vi "carwash_test2_mod.vi"() -> ()   [LabVIEW 2017]
panel:
  out "Enum":enum16{""}(ring)
  out "number":u32
  out "x+y":i32
  out "x*y":i32
  out "output cluster":cluster{bool, bool}
  in  "Economy Wash":bool
  in  "Deluxe Wash":bool
  in  "?":bool
  in  "Wash Select":enum16{"Initialize", "Deluxe", "Economy"}(ring)
  out "Vehicle Out of Position":bool=TRUE
  out "Air Dry":bool
  out "Clear Water Rinse":bool
  out "Main High Press. Wash":bool
  out "Soap Application":bool
  out "Under body Wash":bool
  in  "?":bool
  in  "0":bool
  in  "stop":bool
  # "Car Wash Indicators"
  # "Underbody wash\nposition \nSwitch"
  # "Main Wash \nPosition \nSwitch"
  # "Air Dry\nPosition\nSwitch"
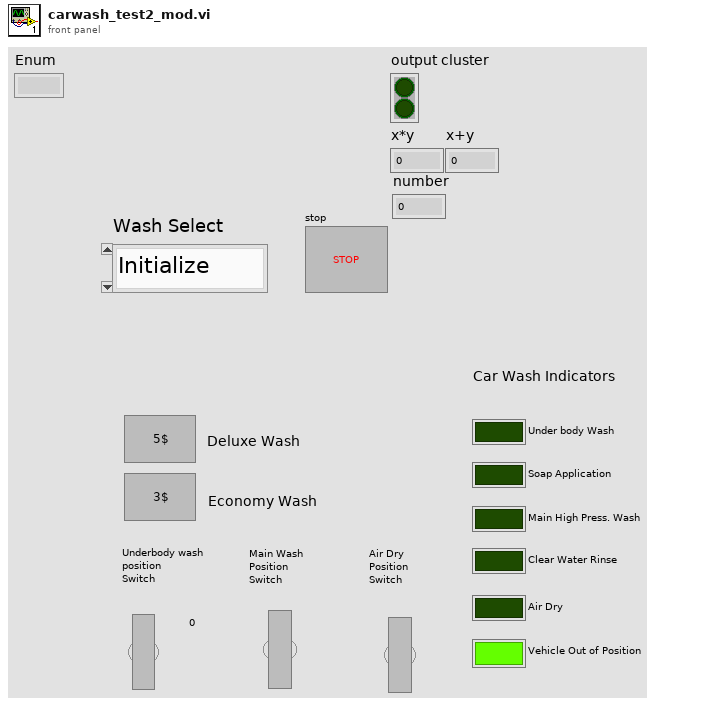
[diagram p1: front panel]
types:
  T1 = enum8{"Enabled", "Disabled", "Disabled and Grayed Out"}
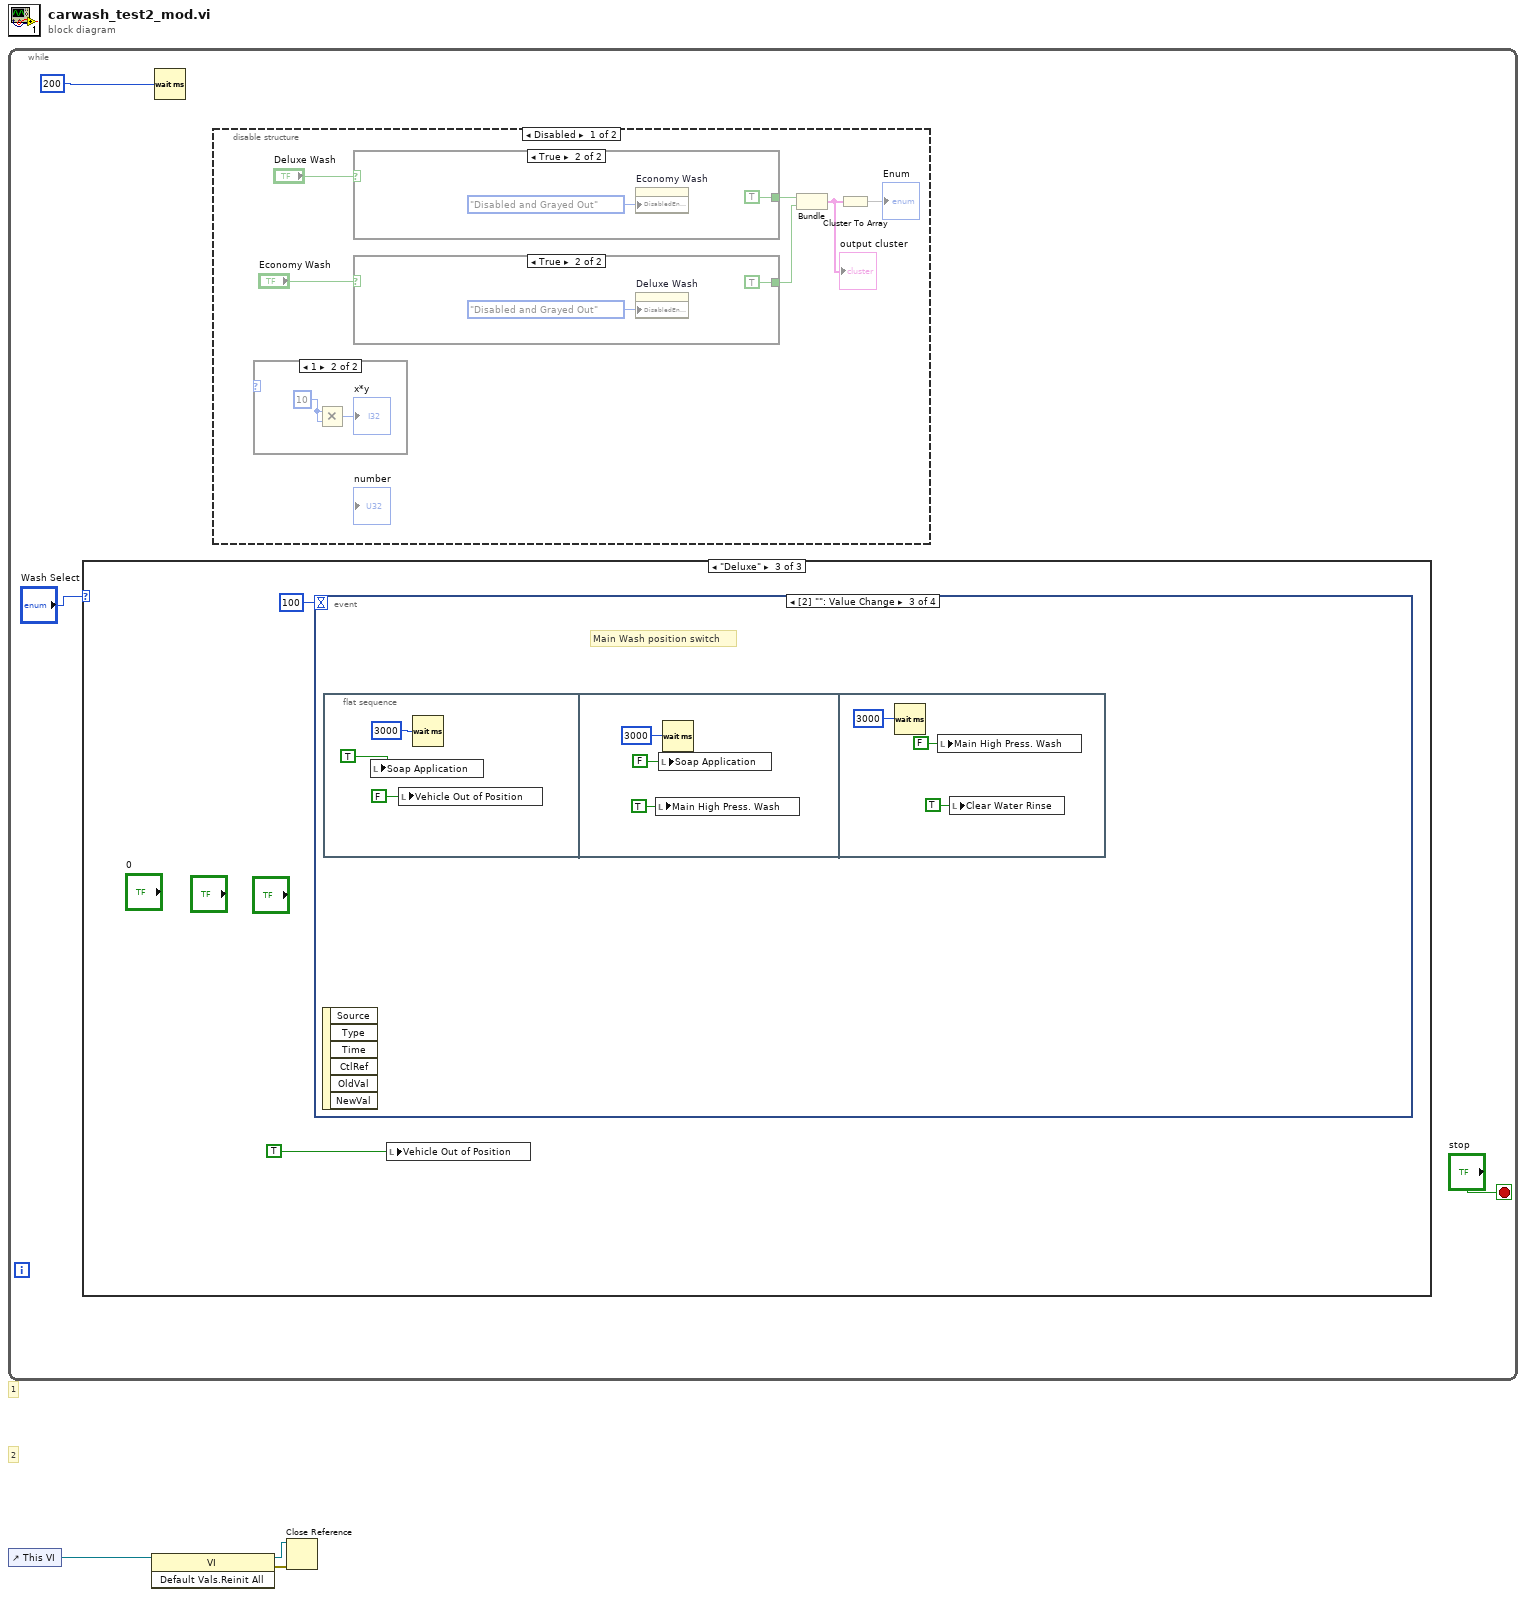
[diagram p0: block diagram]
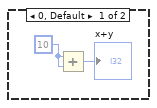
[diagram p2: hidden frame]
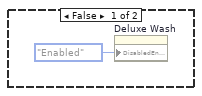
[diagram p3: hidden frame]
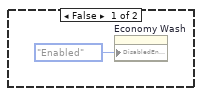
[diagram p4: hidden frame]
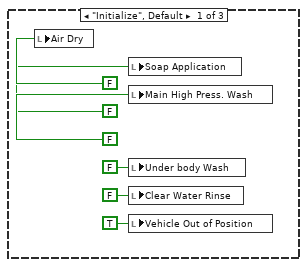
[diagram p6: hidden frame]
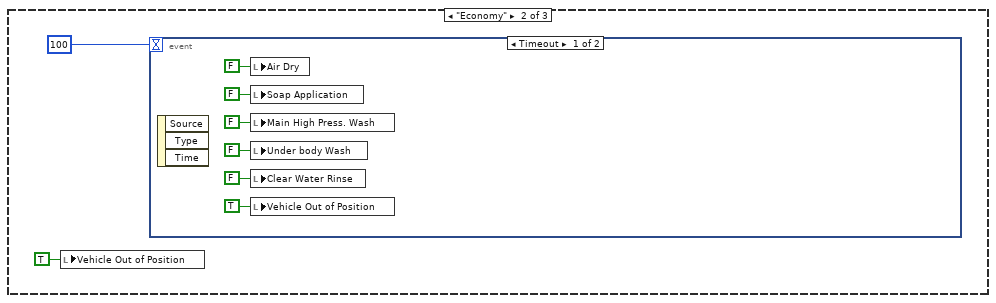
[diagram p7: hidden frame]
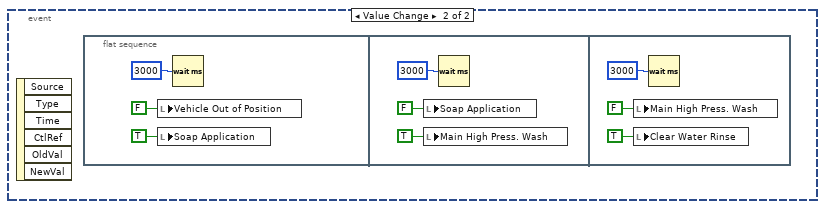
[diagram p8: hidden frame]
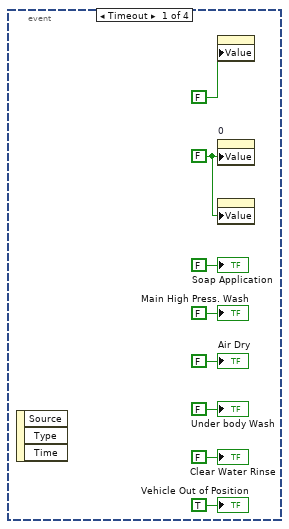
[diagram p9: hidden frame]
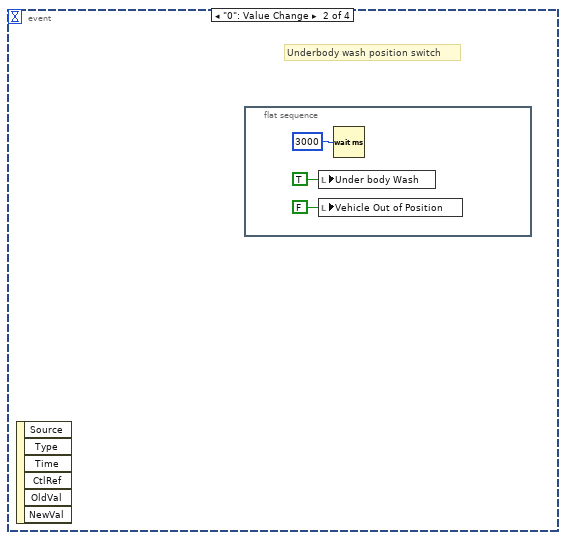
[diagram p10: hidden frame]
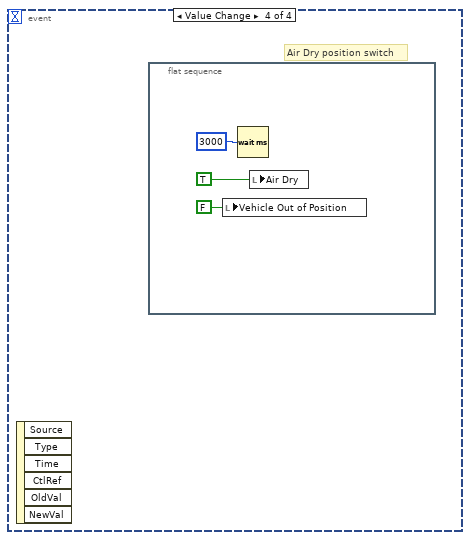
[diagram p11: hidden frame]
diagram:
  # "1"
  # "2"
  n1 = while {
    stop <- "stop" stop-if-true
    n2 = case shown="\"Deluxe\"" "Wash Select" {
      frame "Initialize", Default {
        n3 = local write "Air Dry"(FALSE) -> ()
        n4 = local write "Soap Application"(FALSE) -> ()
        n5 = local write "Main High Press. Wash"(FALSE) -> ()
        n6 = local write "Under body Wash"(FALSE) -> ()
        n7 = local write "Clear Water Rinse"(FALSE) -> ()
        n8 = local write "Vehicle Out of Position"(TRUE) -> ()
      }
      frame "Economy" {
        n9 = local write "Vehicle Out of Position"(TRUE ("Vehicle Out of Position")) -> ()
        n10 = event shown="[0] Timeout" {
          selector: _ -> [_ _]
          dyn-events: _ -> [_ _]
          timeout: 100 -> [_ _]
          event Timeout {
            n11 = event-data() -> ()  [unwired: 1 in, 3 out]
            n12 = local write "Air Dry"(FALSE) -> ()
            n13 = local write "Soap Application"(FALSE) -> ()
            n14 = local write "Main High Press. Wash"(FALSE) -> ()
            n15 = local write "Under body Wash"(FALSE) -> ()
            n16 = local write "Clear Water Rinse"(FALSE) -> ()
            n17 = local write "Vehicle Out of Position"(TRUE ("Vehicle Out of Position")) -> ()
          }
          event Value Change {
            n18 = event-data() -> ()  [unwired: 1 in, 6 out]
            n19 = flat-sequence {
              frame #0 {
                n20 = local write "Vehicle Out of Position"(FALSE ("Vehicle Out of Position")) -> ()
                n21 = local write "Soap Application"(TRUE ("Soap Application")) -> ()
                n22 = Wait (ms)(milliseconds to wait=u32 3000) -> ()  [unwired: 1 out]
              }
              frame #1 {
                n23 = local write "Soap Application"(FALSE ("Soap Application")) -> ()
                n24 = local write "Main High Press. Wash"(TRUE ("Main High Press. Wash")) -> ()
                n25 = Wait (ms)(milliseconds to wait=u32 3000) -> ()  [unwired: 1 out]
              }
              frame #2 {
                n26 = local write "Main High Press. Wash"(FALSE ("Main High Press. Wash")) -> ()
                n27 = local write "Clear Water Rinse"(TRUE ("Clear Water Rinse")) -> ()
                n28 = Wait (ms)(milliseconds to wait=u32 3000) -> ()  [unwired: 1 out]
              }
            }
          }
        }
      }
      frame "Deluxe" {
        n29 = event shown="[2] \"\": Value Change" {
          selector: _ -> [_ _ _ _]
          dyn-events: _ -> [_ _ _ _]
          timeout: 100 -> [_ _ _ _]
          event Timeout {
            w55 = FALSE
            n30 = event-data() -> ()  [unwired: 1 in, 3 out]
            n31 = property class="Bool (strict)"("Value"=FALSE) -> ()  [unwired: 2 in, 2 out]
            n32 = property on="0" class="Bool (strict)"("Value"=w55) -> ()  [unwired: 2 in, 2 out]
            n33 = property class="Bool (strict)"("Value"=w55) -> ()  [unwired: 2 in, 2 out]
            "Air Dry" <- FALSE
            "Vehicle Out of Position" <- TRUE
            "Clear Water Rinse" <- FALSE
            "Under body Wash" <- FALSE
            "Main High Press. Wash" <- FALSE
            "Soap Application" <- FALSE
          }
          event "0": Value Change {
            # "Underbody wash position switch"
            n34 = event-data() -> ()  [unwired: 1 in, 6 out]
            n35 = flat-sequence {
              frame #0 {
                n36 = local write "Under body Wash"(TRUE ("Under body Wash")) -> ()
                n37 = local write "Vehicle Out of Position"(FALSE ("Vehicle Out of Position")) -> ()
                n38 = Wait (ms)(milliseconds to wait=u32 3000) -> ()  [unwired: 1 out]
              }
            }
          }
          event Value Change {
            # "Main Wash position switch"
            n39 = event-data() -> ()  [unwired: 1 in, 6 out]
            n40 = flat-sequence {
              frame #0 {
                n41 = local write "Soap Application"(TRUE ("Air Dry")) -> ()
                n42 = local write "Vehicle Out of Position"(FALSE ("Vehicle Out of Position")) -> ()
                n43 = Wait (ms)(milliseconds to wait=u32 3000) -> ()  [unwired: 1 out]
              }
              frame #1 {
                n44 = local write "Main High Press. Wash"(TRUE ("Main High Press. Wash")) -> ()
                n45 = local write "Soap Application"(FALSE ("Under body Wash")) -> ()
                n46 = Wait (ms)(milliseconds to wait=u32 3000) -> ()  [unwired: 1 out]
              }
              frame #2 {
                n47 = Wait (ms)(milliseconds to wait=u32 3000) -> ()  [unwired: 1 out]
                n48 = local write "Main High Press. Wash"(FALSE ("Main High Press. Wash")) -> ()
                n49 = local write "Clear Water Rinse"(TRUE ("Clear Water Rinse")) -> ()
              }
            }
          }
          event Value Change {
            # "Air Dry position switch"
            n50 = event-data() -> ()  [unwired: 1 in, 6 out]
            n51 = flat-sequence {
              frame #0 {
                n52 = local write "Vehicle Out of Position"(FALSE ("Vehicle Out of Position")) -> ()
                n53 = Wait (ms)(milliseconds to wait=u32 3000) -> ()  [unwired: 1 out]
                n54 = local write "Air Dry"(TRUE ("Boolean 2")) -> ()
              }
            }
          }
        }
        n55 = local write "Vehicle Out of Position"(TRUE ("Vehicle Out of Position")) -> ()
      }
    }
    n56 = Wait (ms)(milliseconds to wait=u32 200) -> ()  [unwired: 1 out]
    n57 = disable-structure shown="Disabled" {
      frame Disabled {
        n58 = case shown="1" {
          selector: _ -> [_ _]
          frame 0, Default {
            w14 = 10
            n59 = Add(x=w14, y=w14) -> (x+y=→"x+y":i32)
          }
          frame 1 {
            w16 = 10
            n60 = Multiply(x=w16, y=w16) -> (x*y=→"x*y":i32)
          }
        }
        n61 = case shown="True" "Deluxe Wash" {
          tunnel: [_ TRUE] -> w10
          frame False {
            n62 = property on="Economy Wash" class="Bool (strict)"("DisabledEnum"=T1."Enabled" ("Disabled")) -> ()  [unwired: 2 in, 2 out]
          }
          frame True {
            n63 = property on="Economy Wash" class="Bool (strict)"("DisabledEnum"=T1."Disabled and Grayed Out" ("Disabled")) -> ()  [unwired: 2 in, 2 out]
          }
        }
        n64 = case shown="True" "Economy Wash" {
          tunnel: [_ TRUE] -> w9
          frame False {
            n65 = property on="Deluxe Wash" class="Bool (strict)"("DisabledEnum"=T1."Enabled" ("Disabled")) -> ()  [unwired: 2 in, 2 out]
          }
          frame True {
            n66 = property on="Deluxe Wash" class="Bool (strict)"("DisabledEnum"=T1."Disabled and Grayed Out" ("Disabled")) -> ()  [unwired: 2 in, 2 out]
          }
        }
        n67 = Bundle(w10, w9) -> (w8:cluster{bool, bool})  [unwired: 1 in]
        "output cluster" <- w8
        n68 = Cluster To Array(cluster=w8) -> (array=→"Enum":bool[])
      }
      frame Enabled {
      }
    }
  }
  n69 = control-ref of="This VI"() -> (w3:refnum<vi>)
  n70 = invoke class="VI" method="Default Vals.Reinit All"(reference=w3) -> (reference out=w2:refnum<vi>, error out=w1:errorcluster)  [unwired: 2 in, 1 out]
  n71 = Close Reference(reference=w2, error in (no error)=w1) -> ()  [unwired: 1 out]
